vi "Scaning - wait_3_4DipoleMagnet.vi"() -> ()   [LabVIEW 2018]
uses:
  <vilib>/userdefined/High Color/nirio_resource_hc.ctl
  <vilib>/LabVIEW Targets/FPGA/cRIO/shared/nicrio_ModuleControls/nicrio_cRIO-9239_DataRatesRing.ctl
  Control 2.ctl
  <vilib>/Platform/TimedLoop/XDataNode/timing_clust.ctl
  <vilib>/Platform/TimedLoop/XDataNode/nitl_modes.ctl
  <vilib>/Platform/TimedLoop/XDataNode/wakeup.ctl
  <vilib>/LabVIEW Targets/FPGA/cRIO/shared/nicrio_ModuleControls/nicrio_calibrationModTypeEnum.ctl
  <vilib>/FPGAPlugInAG/cRIO-9054/niLvFpga_Open_cRIO-9054.vi
  <vilib>/rvi/interface/common/dynamic/niFpgaDynamicAddResources.vi
  <vilib>/FPGAPlugInAG/Dynamic/niLvFpga_Reset_Dynamic.vi
  <vilib>/Utility/error.llb/Error Cluster From Error Code.vi
  <vilib>/rvi/errors/niLvFpgaAdjustHostInterfaceError.vi
  <vilib>/FPGAPlugInAG/Dynamic/niLvFpga_Run_Dynamic.vi
  calab/vis/Private/Put_DBL-1D_PV-1D.vi
  <vilib>/FPGAPlugInAG/Dynamic/niLvFpga_Close_Dynamic.vi
  calab/vis/Private/Get_PV.vi
  calab/vis/Private/Put_DBL_PV.vi
  <vilib>/rvi/interface/nirviOpenFPGA/nirviOpenFPGA.xnode
  FPGA Bitfiles/9239_FPGATarget_NI9239GettingSta_jF2totIdoNE.lvbitx
  <vilib>/rvi/interface/nirviMethod/nirviMethod.xnode
  <vilib>/rvi/interface/nirviReadWriteControl/nirviReadWriteControl.xnode
  <vilib>/platform/TimedLoop/XDataNode/XDataNode.xnode
  <vilib>/rvi/interface/nirviCloseFPGA/nirviCloseFPGA.xnode
  NiFpgaLv.dll
  <vilib>/rvi/interface/Simulation/niFpgaSimulationCallBeginRW.vi
  <vilib>/FPGAPlugInAG/Dynamic/niLvFpga_ReadFifo_Dynamic.vi
  <vilib>/rvi/errors/niLvFpgaMergeErrorWithErrorCode.vi
  <vilib>/Platform/TimedLoop/XDataNode/XDNodeRunTimeDep.lvlib
  calab/vis/Private/Put_Boolean-1D_PV.vi
panel:
  in  "Current_Set":dbl=360.0 format="%#_13g"
  in  "1234":bool
  in  "34":bool
  in  "12":bool
  in  "CurrentRateSet A/s":dbl=1.0 format="%#_13g"
  in  "Range":dbl
  in  "本底":sgl
  out "size(s)":i32
  in  "Data Rate 2":u8
  in  "Period":i64=20
  out "Appended path":path=path "/home/lvuser/natinst/bin/20250919-2data"
  in  "保存数据?":bool
  in  "Save data":string="20250919-2"
  in  "Wait Times":dbl=2.0
  in  "Wait Step":dbl=10.0
  out "磁铁电流/A":sgl(graph)
  out "FC电流/nA":sgl(graph)
  in  "Current_Stop":dbl=120.0 format="%#_13g"
  in  "Current_Start":dbl=25.0 format="%#_13g"
  out "Elements Remaining 2":u32
  out "Current":cluster{"X":sgl, "Y":sgl}[](graph)
  in  "Data Rate":T1=5 items=["50.000 kS/s (NI 9239)"=1, "25.000 kS/s (NI 9239)"=2, "16.667 kS/s (NI 9239)"=3, "12.500 kS/s (NI 9239)"=4, "10.000 kS/s (NI 9239)"=5, "8.333 kS/s (NI 9239)"=6, "7.143 kS/s (NI 9239)"=7, "6.250 kS/s (NI 9239)"=8, "5.556 kS/s (NI 9239)"=9, "5.000 kS/s (NI 9239)"=10, "4.545 kS/s (NI 9239)"=11, "4.167 kS/s (NI 9239)"=12, "3.846 kS/s (NI 9239)"=13, "3.571 kS/s (NI 9239)"=14, "3.333 kS/s (NI 9239)"=15, "3.125 kS/s (NI 9239)"=16, "2.941 kS/s (NI 9239)"=17, "2.778 kS/s (NI 9239)"=18, "2.632 kS/s (NI 9239)"=19, "2.500 kS/s (NI 9239)"=20, "2.381 kS/s (NI 9239)"=21, "2.273 kS/s (NI 9239)"=22, "2.174 kS/s (NI 9239)"=23, "2.083 kS/s (NI 9239)"=24, "2.000 kS/s (NI 9239)"=25, "1.923 kS/s (NI 9239)"=26, "1.852 kS/s (NI 9239)"=27, "1.786 kS/s (NI 9239)"=28, "1.724 kS/s (NI 9239)"=29, "1.667 kS/s (NI 9239)"=30, "1.613 kS/s (NI 9239)"=31]
  out "Host error out":errorcluster
  out "FPGA error out":errorcluster
  in  "stop":bool
  out "Data FIFO Full":bool
  in  "Start":bool
  in  "AVG":bool=TRUE
  in  "ave_num":u8=200
  in  "RIO Device":T2="RIO0"
  # "A"
  # "A"
  # "秒"
  # "A"
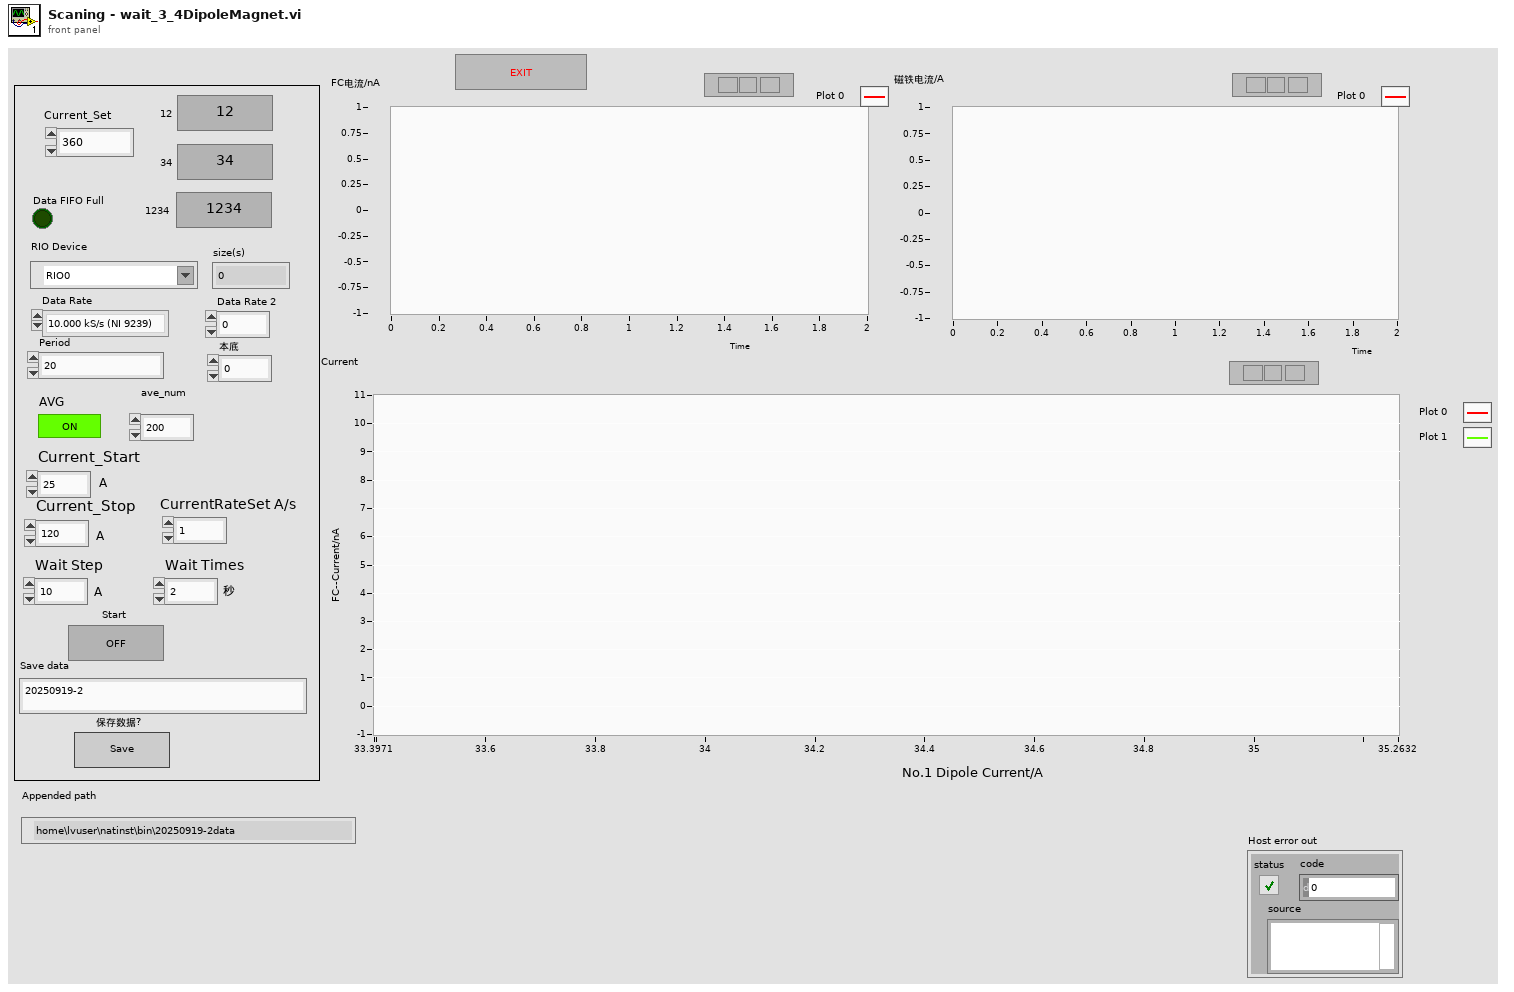
[diagram p1: front panel]
types:
  T1 = typedef "nicrio_cRIO-9239_DataRatesRing.ctl" = u8
  T2 = typedef "nirio_resource_hc.ctl" = tag
  T3 = enum16{"open", "replace", "create", "open or create", "replace or create", "replace or create with confirmation"}
  T4 = typedef "Control 2.ctl" = enum16{"idel", "Scaning", "SetHV", "SetHV2", "Wait", ""}
  T5 = typedef "XDNodeRunTimeDep.lvlib/timing_clust.ctl" = cluster{"Expected End [f-1]":u64, "Actual End [f-1]":u64, "Finished Late? [f-1]":bool, "Expected End [i-1]":u64, "Actual End [i-1]":u64, "Finished Late? [i-1]":bool, "Expected Start [i]":u64, "Actual Start [i]":u64, "Expected Start [f]":u64, "Actual Start [f]":u64, "Source Name":string, "Structure Name":string, "Period":i64, "Deadline":i64, "Offset":i64, "Start":i64, "Priority":i32, "Timeout":i32, "Mode":T6, "Wakeup Reason":T7, "Error":errorcluster, "Source Type":string, "Secondary Source Type":string, "Global End Time":u64, "Global Start Time":u64, "Frame Duration":u64, "Iteration Duration":u64, "Assigned CPU":i32, "I/O Scan Engine Mode":u32}
  T6 = typedef "XDNodeRunTimeDep.lvlib/nitl_modes.ctl" = enum32{"No Change", "Process missed periods, maintain original phase", "Discard missed periods, maintain original phase", "Process missed periods, ignore original phase", "Discard missed periods, ignore original phase"}
  T7 = typedef "XDNodeRunTimeDep.lvlib/wakeup.ctl" = enum32{"Normal", "Aborted", "Asynchronous wakeup", "Timing source error", "Timed loop error", "Timeout"}
  T8 = enum16{"big-endian, network order", "native, host order", "little-endian"}
  T9 = typedef "nicrio_calibrationModTypeEnum.ctl" = enum8{"NI 9201", "NI 9203 (4-20 mA range)", "NI 9203 (+/- 20 mA range)", "NI 9205", "NI 9206", "NI 9215", "NI 9221", "NI 9229", "NI 9233", "NI 9234", "NI 9237", "NI 9239", "NI 9263", "NI 9264", "NI 9265", "NI 9217", "NI 9236", "NI 9235", "NI 9225", "NI 9227", "NI 9269", "NI 9222", "NI 9223", "NI 9232", "NI 9381 (AI)", "NI 9381 (AO)", "NI 9220", "NI 9238", "NI 9218 (+/- 60 V range)", "NI 9218 (+/- 16 V range)", "NI 9218 (+/- 65 mV range)", "NI 9218 (+/- 5V IEPE range)", "NI 9218 (+/- 20 mA range)", "NI 9218 (+/- 22 mV/V range)", "NI 9260", "NI 9216", "NI 9226", "NI 9246", "NI 9247", "NI 9230", "NI 9266", "Ni 9775  (AI)", "NI 9775 (Trigger Level)", "NI 9775 (Hysteresis Level)", "NI 9684 (+/- 10 V range)", "NI 9684 (+/- 5 V range)"}
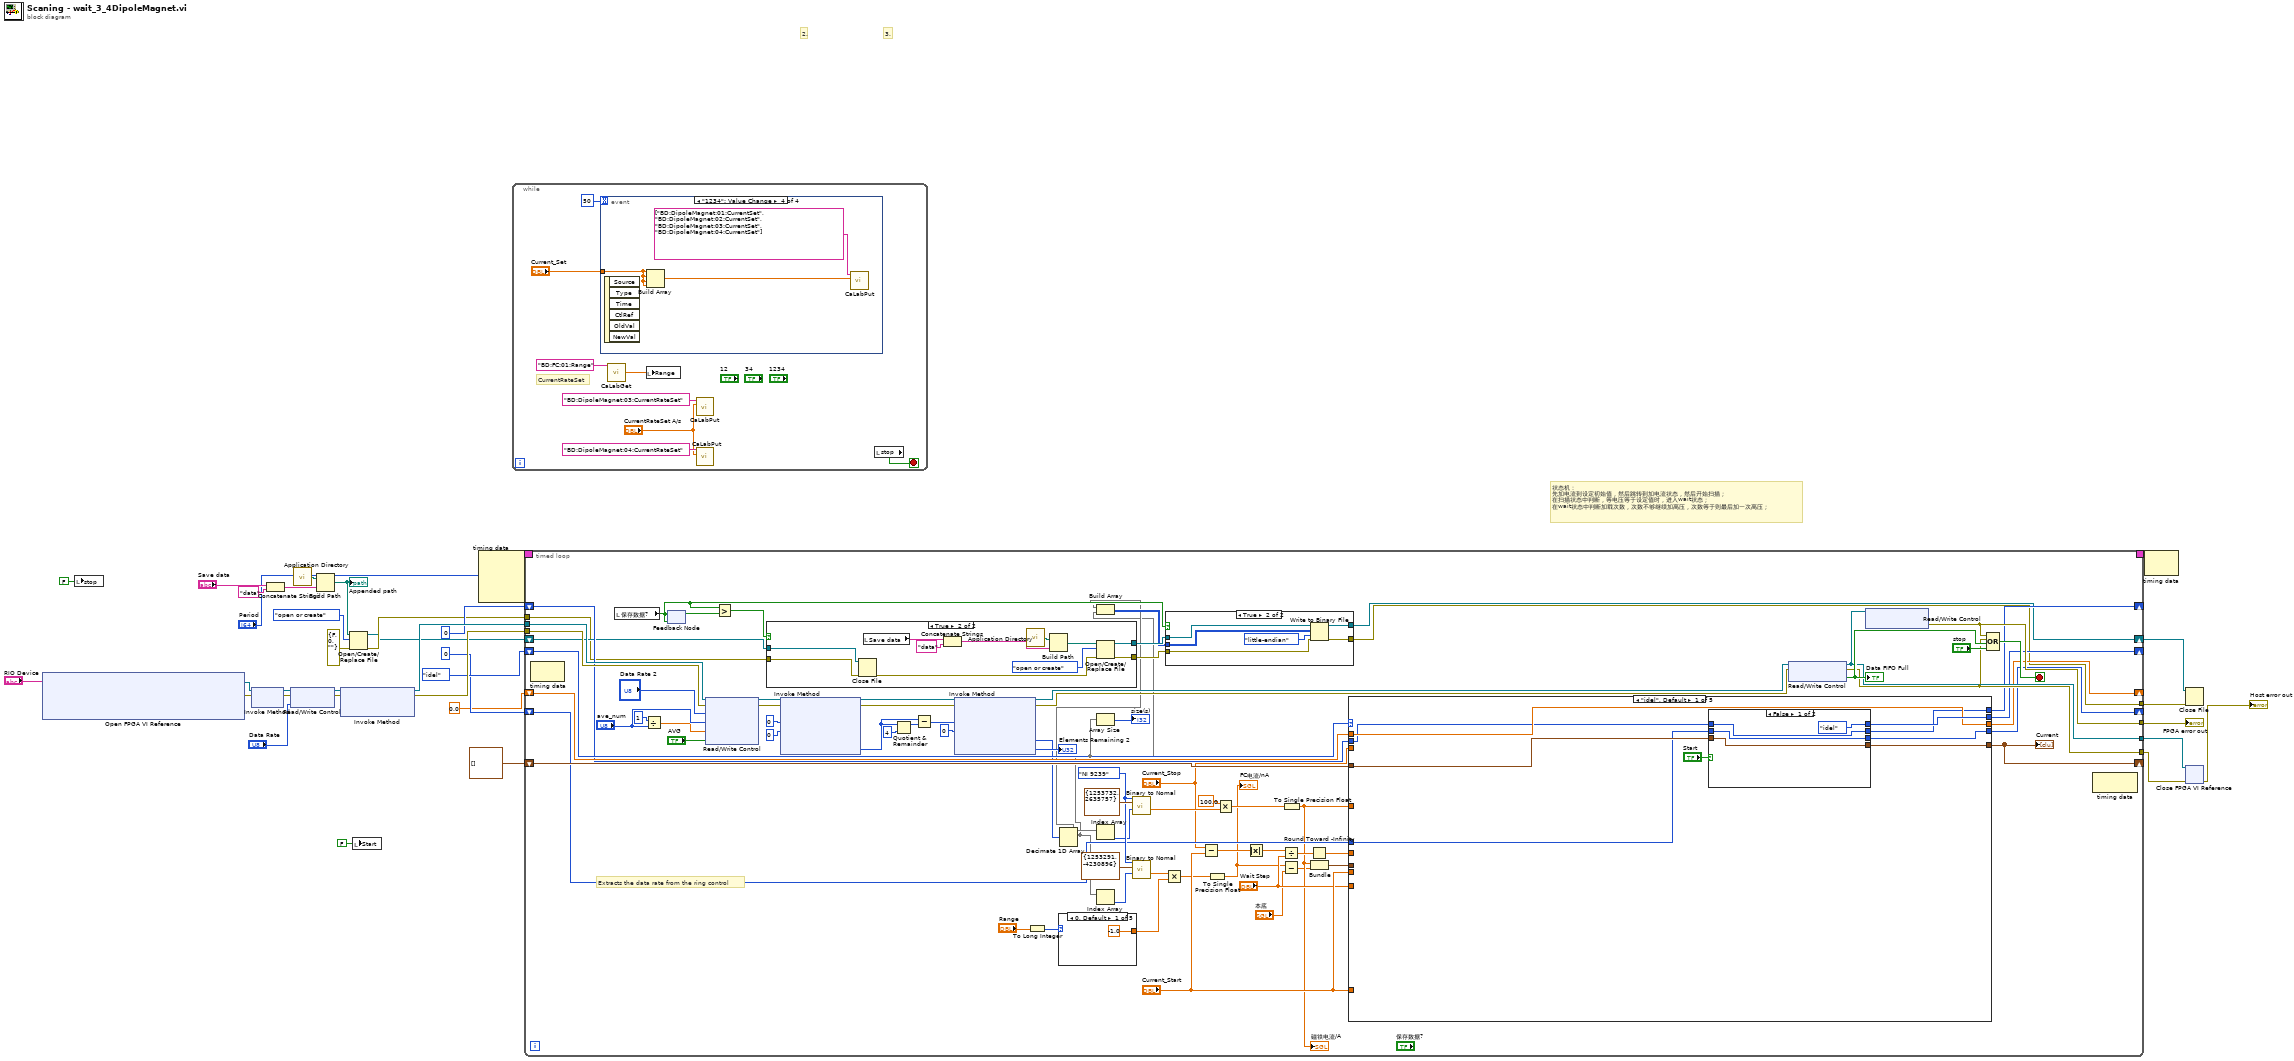
[diagram p0: block diagram]
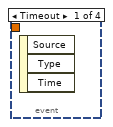
[diagram p2: hidden frame]
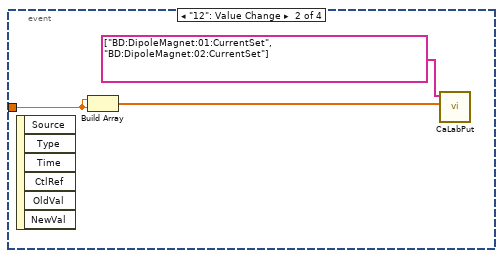
[diagram p3: hidden frame]
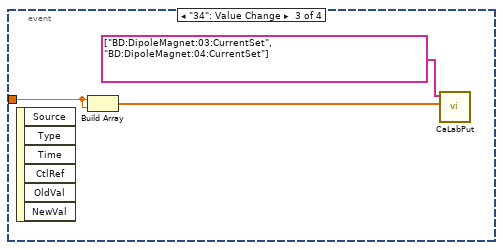
[diagram p4: hidden frame]
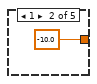
[diagram p5: hidden frame]
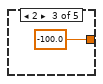
[diagram p6: hidden frame]
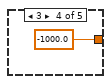
[diagram p7: hidden frame]
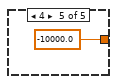
[diagram p8: hidden frame]
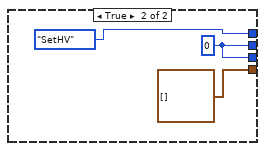
[diagram p11: hidden frame]
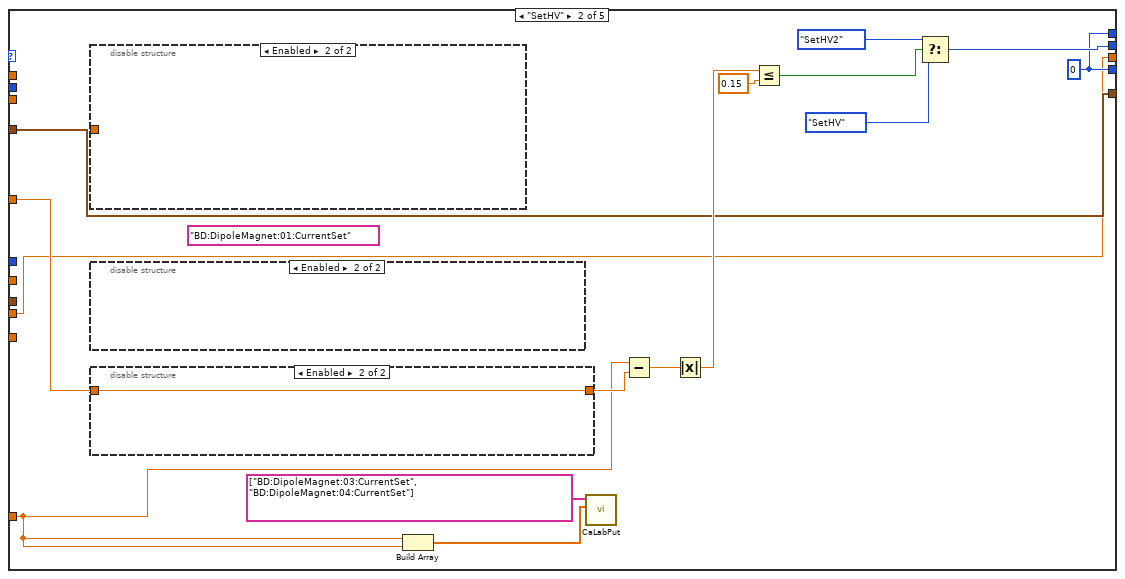
[diagram p12: hidden frame]
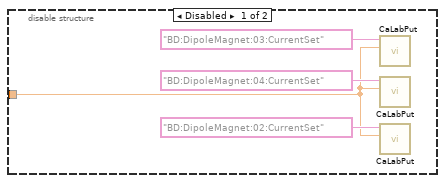
[diagram p13: hidden frame]
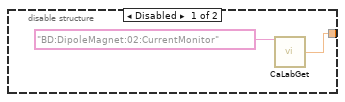
[diagram p14: hidden frame]
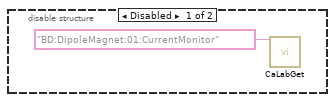
[diagram p15: hidden frame]
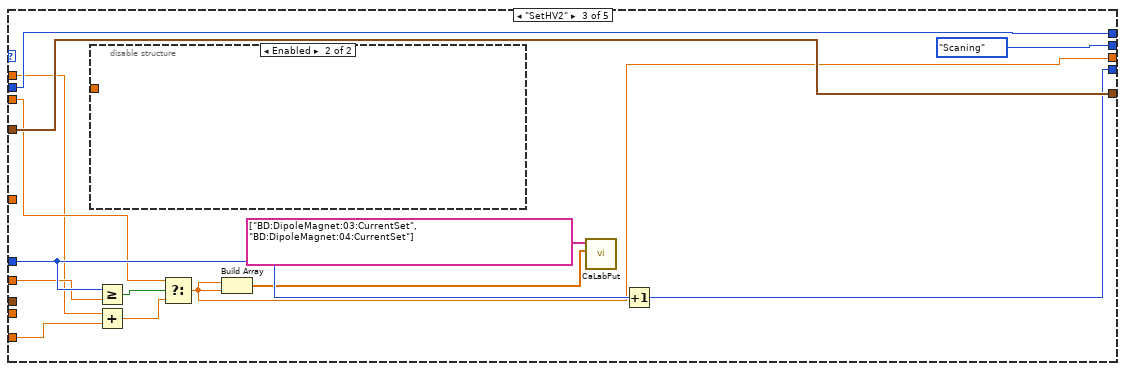
[diagram p16: hidden frame]
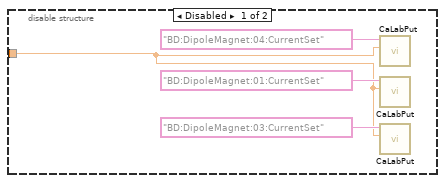
[diagram p17: hidden frame]
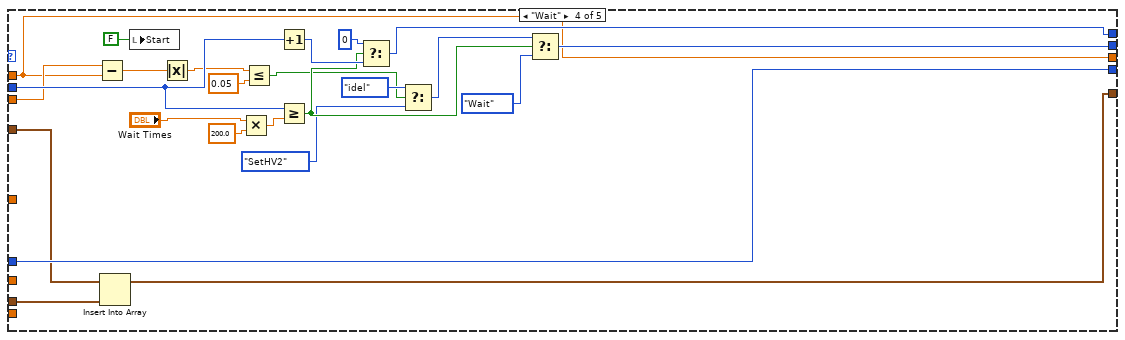
[diagram p18: hidden frame]
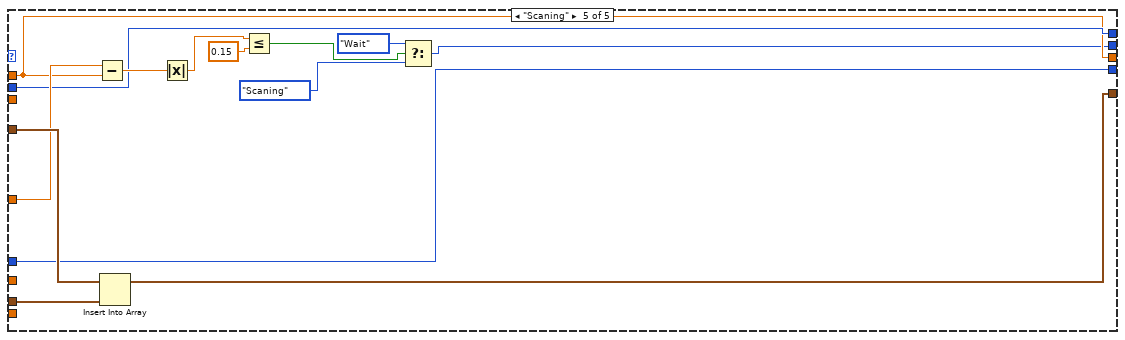
[diagram p19: hidden frame]
diagram:
  # "状态机：\n先加电流到设定初始值，然后跳转到加电流状态，然后开始扫描；\n在扫描状态中判断，等电压等于设定值时，进入wait状态；\n在wait状态中判断加载次数，次数不够继续加高压，次数等于则最后加一次高压；"
  # "3."
  # "2."
  n1 = xnode "Open FPGA VI Reference"("resource name"="RIO Device") -> ("FPGA VI Reference Out"=w27:refnum<k20>, "error out"=w23:errorcluster)  [unwired: 1 in]
  n2 = local write "stop"(FALSE ("stop")) -> ()
  n3 = xnode "Invoke Method"("FPGA VI Reference In"=w27, "error in"=w23) -> ("FPGA VI Reference Out"=w26:refnum<k20>, "error out"=w28:errorcluster)
  n4 = Concatenate Strings("Save data", "data" ("string")) -> (w12:string)
  n5 = xnode "Read/Write Control"("FPGA VI Reference In"=w26, "error in"=w28, "Data Rate"="Data Rate") -> ("FPGA VI Reference Out"=w31:refnum<k20>, "error out"=w32:errorcluster)
  n6 = call <vilib>:"Application Directory.vi"() -> ("Application Directory"=w15:path)
  n7 = Build Path(base path=w15, name or relative path=w12) -> (appended path=w16:path)
  "Appended path" <- w16
  n8 = xnode "Invoke Method"("FPGA VI Reference In"=w31, "error in"=w32) -> ("FPGA VI Reference Out"=w34:refnum<k20>, "error out"=w35:errorcluster)  [unwired: 1 in]
  n9 = Open/Create/Replace File(file path (use dialog)=w16, error in=errorcluster {"status"=FALSE, "code"=0, "source"=""}, operation (0:open)=T3."open or create") -> (refnum out=w8:refnum<file>, error out=w10:errorcluster)  [unwired: 3 in, 1 out]
  n10 = local write "Start"(FALSE ("Start")) -> ()
  n11 = node-c288("Period") -> (w5:T5)  [unwired: 3 in]
  n12 = while {
    stop <- w42 stop-if-true
    # "CurrentRateSet"
    n13 = event shown="[3] \"1234\": Value Change" {
      selector: _ -> [_ _ _ _]
      dyn-events: _ -> [_ _ _ _]
      timeout: 50 -> [_ _ _ _]
      tunnel: "Current_Set" -> [_ w45 w48 w51]
      event Timeout {
        n14 = event-data() -> ()  [unwired: 1 in, 3 out]
      }
      event "12": Value Change {
        n15 = event-data() -> ()  [unwired: 1 in, 6 out]
        n16 = Build Array(w45, w45) -> (w44:dbl[])
        n17 = call-poly "CaLabPut.vi"("Values"=w44, "PV Names"=string[] ["BD:DipoleMagnet:01:CurrentSet", "BD:DipoleMagnet:02:CurrentSet"]) -> ()  [unwired: 6 in, 4 out]
      }
      event "34": Value Change {
        n18 = event-data() -> ()  [unwired: 1 in, 6 out]
        n19 = Build Array(w48, w48) -> (w47:dbl[])
        n20 = call-poly "CaLabPut.vi"("Values"=w47, "PV Names"=string[] ["BD:DipoleMagnet:03:CurrentSet", "BD:DipoleMagnet:04:CurrentSet"]) -> ()  [unwired: 6 in, 4 out]
      }
      event "1234": Value Change {
        n21 = event-data() -> ()  [unwired: 1 in, 6 out]
        n22 = Build Array(w51, w51, w51, w51) -> (w50:dbl[])
        n23 = call-poly "CaLabPut.vi"("Values"=w50, "PV Names"=string[] ["BD:DipoleMagnet:01:CurrentSet", "BD:DipoleMagnet:02:CurrentSet", "BD:DipoleMagnet:03:CurrentSet", "BD:DipoleMagnet:04:CurrentSet"]) -> ()  [unwired: 6 in, 4 out]
      }
    }
    n24 = call-poly "CaLabGet.vi"("PV Name"="BD:FC:01:Range") -> ("1rst Value (number)"=w41:dbl)  [unwired: 8 in, 6 out]
    n25 = local write "Range"(w41) -> ()
    n26 = call-poly "CaLabPut.vi"("Value"="CurrentRateSet A/s", "PV Name"="BD:DipoleMagnet:03:CurrentRateSet") -> ()  [unwired: 6 in, 4 out]
    n27 = call-poly "CaLabPut.vi"("Value"="CurrentRateSet A/s", "PV Name"="BD:DipoleMagnet:04:CurrentRateSet") -> ()  [unwired: 6 in, 4 out]
    n28 = local read "stop"() -> (w42:bool)
  }
  n29 = timed-loop {
    tunnel: w35 -> [w119]
    tunnel: w34 -> [w120]
    tunnel: [w125] -> w33
    tunnel: [w124] -> w30
    tunnel: [w123] -> w24
    shift-right: [w121] -> _
    shift-left: Control_2."idel" -> [w122]
    shift-right: [w60] -> _
    shift-left: cluster{"X":sgl, "Y":sgl}[] [] ("XY Graph") -> [w113]
    shift-right: [w92] -> _
    shift-left: 0 -> [w99]
    shift-right: [w90] -> _
    shift-left: 0.0 -> [w91]
    shift-right: [w87] -> _
    shift-left: 0 -> [w88]
    tunnel: w10 -> [w74]
    tunnel: [w72] -> w7
    shift-right: [w70] -> w6
    shift-left: w8 -> [w75]
    timing: w5 -> [_]
    timing-out: [_] -> w4
    stop <- w128 stop-if-true
    w111 = nicrio_calibrationModTypeEnum."NI 9239" ("Module Type")
    # "Extracts the data rate from the ring control"
    n30 = node-c288() -> ()  [unwired: 1 in, 1 out]
    n31 = local read "保存数据?"() -> (w77:bool)
    n32 = Divide(x=u8 1, y="ave_num") -> (x/y=w114:dbl)
    n33 = feedback #1(w77) -> (w76:bool)
    n34 = feedback-in #1(w77) -> ()
    n35 = xnode "Read/Write Control"("FPGA VI Reference In"=w120, "error in"=w119, "Period(uSec)"="Data Rate 2", "ave_num"="ave_num", "1/num"=w114, "AVG"="AVG") -> ("FPGA VI Reference Out"=w106:refnum<k20>, "error out"=w107:errorcluster)
    n36 = Greater?(x=w77, y=w76) -> (0:w78:bool)
    n37 = case shown="True" w78 {
      tunnel: w75 -> [w137 w148]
      tunnel: w74 -> [w136 w147]
      tunnel: [w137 w140] -> w79
      tunnel: [w136 w139] -> w73
      frame False {
      }
      frame True {
        n38 = Close File(refnum=w148, error in=w147) -> (error out=w141:errorcluster)  [unwired: 1 out]
        n39 = local read "Save data"() -> (w138:string)
        n40 = Concatenate Strings(w138, "data" ("string")) -> (w146:string)
        n41 = call <vilib>:"Application Directory.vi"() -> ("Application Directory"=w144:path)
        n42 = Build Path(base path=w144, name or relative path=w146) -> (appended path=w145:path)
        n43 = Open/Create/Replace File(file path (use dialog)=w145, error in=w141, operation (0:open)=T3."open or create") -> (refnum out=w140:refnum<file>, error out=w139:errorcluster)  [unwired: 3 in, 1 out]
      }
    }
    n44 = xnode "Invoke Method"("FPGA VI Reference In"=w106, "error in"=w107, "Number of Elements"=u32 0, "Timeout (ms)"=0) -> ("FPGA VI Reference Out"=w82:refnum<k20>, "error out"=w81:errorcluster, "Elements Remaining"=w83:u32)  [unwired: 1 out]
    n45 = Quotient & Remainder(x=w83, y=u32 4) -> (x-y*floor(x/y)=w84:u32)  [unwired: 1 out]
    n46 = Subtract(x=w83, y=w84) -> (x-y=w80:u32)
    n47 = xnode "Invoke Method"("FPGA VI Reference In"=w82, "error in"=w81, "Number of Elements"=w80, "Timeout (ms)"=0 ("Timeout")) -> ("FPGA VI Reference Out"=w105:refnum<k20>, "error out"=w104:errorcluster, "Data"=w69:i32[], "Elements Remaining"=→"Elements Remaining 2":u32)
    n48 = To Long Integer(number="Range") -> (32bit integer=w54:i32)
    n49 = case shown="0, Default" w54 {
      tunnel: [-1.0 ("y") -10.0 ("y") -100.0 ("y") -1000.0 ("y") -10000.0 ("y")] -> w53
      frame 0, Default {
      }
      frame 1 {
      }
      frame 2 {
      }
      frame 3 {
      }
      frame 4 {
      }
    }
    n50 = Decimate 1D Array(w69) -> (w66:i32[], w63:i32[])  [unwired: 2 out]
    n51 = Array Size(array=w63) -> (size(s)=→"size(s)":i32)
    n52 = Index Array(array=w66) -> (element=w65:i32)  [unwired: 1 in]
    n53 = Index Array(array=w63) -> (element=w64:i32)  [unwired: 1 in]
    n54 = Build Array(w66, w63) -> (w71:i32[][])
    n55 = call "Binary to Nomal.vi"("Module Type"=w111, "Channel Calibration"=cluster{"LSB Weight":u32, "Offset":i32} {"LSB Weight"=1253732, "Offset"=2635757}, "Numeric"=w65) -> ("data"=w101:dbl)  [unwired: 11 in, 1 out]
    n56 = call "Binary to Nomal.vi"("Module Type"=w111, "Channel Calibration"=cluster{"LSB Weight":u32, "Offset":i32} {"LSB Weight"=1253291, "Offset"=-4230896} ("Cluster1 2"), "Numeric"=w64) -> ("data"=w100:dbl)  [unwired: 11 in, 1 out]
    n57 = case shown="True" w77 {
      tunnel: [w150 w156] -> w70
      tunnel: w79 -> [w150 w155]
      tunnel: w73 -> [w149 w153]
      tunnel: [w149 w152] -> w72
      tunnel: w71 -> [_ w151]
      frame False {
      }
      frame True {
        n58 = Write to Binary File(file (use dialog)=w155, data=w151, error in=w153, 9:T8."little-endian" ("byte order (0:big-endian, network order)")) -> (refnum out=w156:refnum<file>, error out=w152:errorcluster)  [unwired: 2 in, 1 out]
      }
    }
    n59 = Multiply(x=w100, y=w53) -> (x*y=w68:dbl)
    n60 = Subtract(x="Current_Stop", y="Current_Start") -> (x-y=w98:dbl)
    n61 = To Single Precision Float(number=w68) -> (single precision float=w58:sgl)
    "FC电流/nA" <- w58
    n62 = Multiply(x=100.0, y=w101) -> (x*y=w67:dbl)
    n63 = Absolute Value(x=w98) -> (abs(x)=w97:dbl)
    n64 = Divide(x=w97, y="Wait Step") -> (x/y=w94:dbl)
    n65 = Subtract(x=w58, y="本底") -> (x-y=w56:sgl)
    n66 = To Single Precision Float(number=w67) -> (single precision float=w59:sgl)
    "磁铁电流/A" <- w59
    n67 = Round Toward -Infinity(1:w94) -> (0:w93:dbl)
    n68 = Bundle(w59, w56) -> (w61:cluster{sgl, sgl})  [unwired: 1 in]
    n69 = case shown="\"idel\", Default" w122 {
      tunnel: [w164 w184 Control_2."Scaning" w221 w238] -> w121
      tunnel: w113 -> [w163 w183 w209 w215 w251]
      tunnel: w61 -> [_ _ _ w216 w250]
      tunnel: [w162 w183 w209 w214 w249] -> w60
      tunnel: "Current_Start" -> [_ w175 _ _ _]
      tunnel: w59 -> [_ w179 _ _ w245]
      tunnel: w99 -> [w160 _ w205 w219 w239]
      tunnel: "Current_Start" -> [_ w176 _ _ _]
      tunnel: "Wait Step" -> [_ _ w207 _ _]
      tunnel: w93 -> [_ _ w204 _ _]
      tunnel: [w159 w177 w206 w219 w239] -> w92
      tunnel: w91 -> [w161 _ w199 w220 w240]
      tunnel: [w161 w176 w197 w220 w240] -> w90
      tunnel: "Current_Stop" -> [_ _ w201 w227 _]
      tunnel: w88 -> [w157 _ w200 w233 w241]
      tunnel: [w158 w177 w200 w231 w241] -> w87
      frame "idel", Default {
        n70 = case shown="False" "Start" {
          tunnel: [Control_2."idel" Control_2."SetHV"] -> w164
          tunnel: [w169 cluster{"X":sgl, "Y":sgl}[] [] ("XY Graph")] -> w162
          tunnel: w163 -> [w169 _]
          tunnel: [w167 w170] -> w159
          tunnel: w160 -> [w167 _]
          tunnel: [w166 w170] -> w158
          tunnel: w157 -> [w166 _]
          frame False {
          }
          frame True {
            w170 = 0
          }
        }
      }
      frame "SetHV" {
        w177 = 0
        (unwired) "BD:DipoleMagnet:01:CurrentSet"
        n71 = disable-structure shown="Enabled" {
          disable-tunnel: _ -> [w188 _]
          frame Disabled {
            n72 = call-poly "CaLabPut.vi"("Values"=w188, "PV Name"="BD:DipoleMagnet:03:CurrentSet") -> ()  [unwired: 6 in, 4 out]
            n73 = call-poly "CaLabPut.vi"("Values"=w188, "PV Name"="BD:DipoleMagnet:04:CurrentSet") -> ()  [unwired: 6 in, 4 out]
            n74 = call-poly "CaLabPut.vi"("Values"=w188, "PV Name"="BD:DipoleMagnet:02:CurrentSet") -> ()  [unwired: 6 in, 4 out]
          }
          frame Enabled {
          }
        }
        n75 = disable-structure shown="Enabled" {
          frame Disabled {
            n76 = call-poly "CaLabGet.vi"("PV Name"="BD:DipoleMagnet:01:CurrentMonitor") -> ()  [unwired: 8 in, 7 out]
          }
          frame Enabled {
          }
        }
        n77 = disable-structure shown="Enabled" {
          disable-tunnel: [w192 w194] -> w182
          disable-tunnel: w179 -> [_ w194]
          frame Disabled {
            n78 = call-poly "CaLabGet.vi"("PV Name"="BD:DipoleMagnet:02:CurrentMonitor") -> ("1rst Value (number)"=w192:dbl)  [unwired: 8 in, 6 out]
          }
          frame Enabled {
          }
        }
        n79 = Build Array(w175, w175) -> (w174:dbl[])
        n80 = call-poly "CaLabPut.vi"("Values"=w174, "PV Names"=string[] ["BD:DipoleMagnet:03:CurrentSet", "BD:DipoleMagnet:04:CurrentSet"]) -> ()  [unwired: 6 in, 4 out]
        n81 = Subtract(x=w175, y=w182) -> (x-y=w187:dbl)
        n82 = Absolute Value(x=w187) -> (abs(x)=w186:dbl)
        n83 = Less Or Equal?(x=w186, y=0.15) -> (x <= y?=w178:bool)
        n84 = Select(t=Control_2."SetHV2", s=w178, f=Control_2."SetHV") -> (s? t:f=w184:T4)
      }
      frame "SetHV2" {
        n85 = disable-structure shown="Enabled" {
          disable-tunnel: _ -> [w210 _]
          frame Disabled {
            n86 = call-poly "CaLabPut.vi"("Values"=w210, "PV Name"="BD:DipoleMagnet:04:CurrentSet") -> ()  [unwired: 6 in, 4 out]
            n87 = call-poly "CaLabPut.vi"("Values"=w210, "PV Name"="BD:DipoleMagnet:01:CurrentSet") -> ()  [unwired: 6 in, 4 out]
            n88 = call-poly "CaLabPut.vi"("Values"=w210, "PV Name"="BD:DipoleMagnet:03:CurrentSet") -> ()  [unwired: 6 in, 4 out]
          }
          frame Enabled {
          }
        }
        n89 = Greater Or Equal?(x=w205, y=w204) -> (x >= y?=w203:bool)
        n90 = Add(x=w199, y=w207) -> (x+y=w202:dbl)
        n91 = Select(t=w201, s=w203, f=w202) -> (s? t:f=w197:dbl)
        n92 = Build Array(w197, w197) -> (w196:dbl[])
        n93 = call-poly "CaLabPut.vi"("Values"=w196, "PV Names"=string[] ["BD:DipoleMagnet:03:CurrentSet", "BD:DipoleMagnet:04:CurrentSet"]) -> ()  [unwired: 6 in, 4 out]
        n94 = Increment(x=w205) -> (x+1=w206:i32)
      }
      frame "Wait" {
        n95 = Subtract(x=w227, y=w220) -> (x-y=w230:dbl)
        n96 = Insert Into Array(array=w215, new element=w216) -> (w214:cluster{"X":sgl, "Y":sgl}[])  [unwired: 1 in]
        n97 = local write "Start"(FALSE ("Start")) -> ()
        n98 = Absolute Value(x=w230) -> (abs(x)=w229:dbl)
        n99 = Multiply(x="Wait Times", y=200.0) -> (x*y=w235:dbl)
        n100 = Less Or Equal?(x=w229, y=0.05) -> (x <= y?=w218:bool)
        n101 = Increment(x=w233) -> (x+1=w232:i32)
        n102 = Greater Or Equal?(x=w233, y=w235) -> (x >= y?=w226:bool)
        n103 = Select(t=0, s=w226, f=w232) -> (s? t:f=w231:i32)
        n104 = Select(t=Control_2."idel", s=w218, f=Control_2."SetHV2") -> (s? t:f=w224:T4)
        n105 = Select(t=w224, s=w226, f=Control_2."Wait") -> (s? t:f=w221:T4)
      }
      frame "Scaning" {
        n106 = Subtract(x=w245, y=w240) -> (x-y=w248:dbl)
        n107 = Insert Into Array(array=w251, new element=w250) -> (w249:cluster{"X":sgl, "Y":sgl}[])  [unwired: 1 in]
        n108 = Absolute Value(x=w248) -> (abs(x)=w247:dbl)
        n109 = Less Or Equal?(x=w247, y=0.15) -> (x <= y?=w244:bool)
        n110 = Select(t=Control_2."Wait", s=w244, f=Control_2."Scaning") -> (s? t:f=w238:T4)
      }
    }
    "Current" <- w60
    n111 = xnode "Read/Write Control"("FPGA VI Reference In"=w105, "error in"=w104) -> ("FPGA VI Reference Out"=w125:refnum<k20>, "error out"=w124:errorcluster, "Data FIFO Full"=w127:bool)
    "Data FIFO Full" <- w127
    n112 = xnode "Read/Write Control"("FPGA VI Reference In"=w125) -> ("FPGA Error Out"=w123:errorcluster)  [unwired: 1 in, 2 out]
    n113 = Compound Arithmetic op=OR(w123, w124, w127, "stop") -> (w128:bool)
    n114 = node-c288() -> ()  [unwired: 1 in, 1 out]
  }
  "FPGA error out" <- w24
  n115 = node-c288(w4) -> ()  [unwired: 1 out]
  n116 = Close File(refnum=w6, error in=w7) -> ()  [unwired: 2 out]
  n117 = xnode "Close FPGA VI Reference"("FPGA VI Reference In"=w33, "error in"=w30) -> ("error out"=→"Host error out":errorcluster)
